vi "数据补传对话框.vi"(11 "数据发送时间":timestamp format="%<%Y/%m/%d %%H:%M:%S>T") -> (2 "布尔":bool, 3 "数据发送时间输出":timestamp)   [LabVIEW 2016]
panel:
  in  "取消":bool
  in  "确定":bool
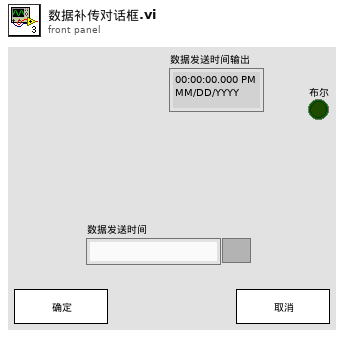
[diagram p1: front panel]
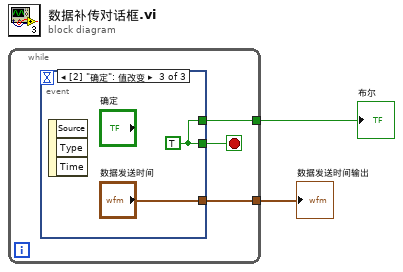
[diagram p0: block diagram]
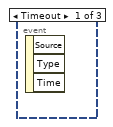
[diagram p2: hidden frame]
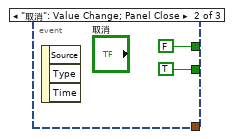
[diagram p3: hidden frame]
diagram:
  n1 = while {
    tunnel: [w4] -> w2
    tunnel: [w3] -> w1
    stop <- w5 stop-if-true
    n2 = event shown="[2] \"确定\": 值改变" {
      selector: _ -> [_ _ _]
      dyn-events: _ -> [_ _ _]
      timeout: _ -> [_ _ _]
      tunnel: [_ TRUE w9] -> w5
      tunnel: [_ FALSE w9] -> w4
      tunnel: [_ _ "数据发送时间"] -> w3
      event Timeout {
        n3 = event-data() -> ()  [unwired: 1 in, 3 out]
      }
      event "取消": Value Change; Panel Close {
        n4 = event-data() -> ()  [unwired: 1 in, 3 out]
      }
      event "确定": Value Change {
        w9 = TRUE
        n5 = event-data() -> ()  [unwired: 1 in, 3 out]
      }
    }
  }
  "布尔" <- w2
  "数据发送时间输出" <- w1
